vi "Recompile_all.vi"   [LabVIEW 2022 SP3]
uses:
  Anemometry Sub Vis/Globals/Constants_global.vi
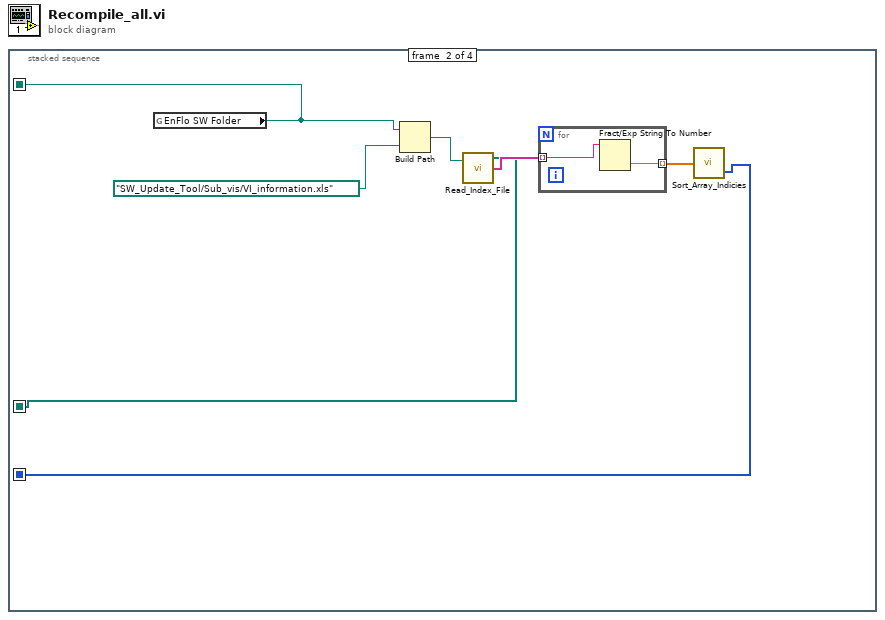
[diagram p0: block diagram]
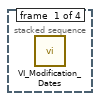
[diagram p2: hidden frame]
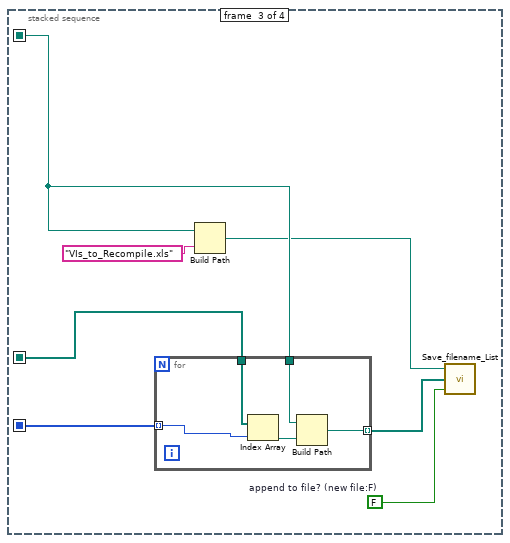
[diagram p3: hidden frame]
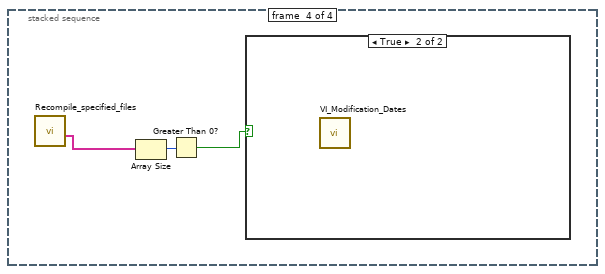
[diagram p4: hidden frame]
diagram:
  n1 = stacked-sequence {
    seq-local: [_ w3 _ _] -> [_ _ w15 _]
    seq-local: [_ w2 _ _] -> [_ _ w14 _]
    seq-local: [_ w1 _ _] -> [_ _ w13 _]
    frame #0 {
      n2 = call "VI_Modification_Dates.vi"() -> ()  [unwired: 1 out]
    }
    frame #1 {
      n3 = global read "Constants_global.vi" "EnFlo SW Folder"() -> (w1:path)
      n4 = Build Path(base path=w1, name or relative path=path "SW_Update_Tool/Sub_vis/VI_information.xls") -> (appended path=w6:path)
      n5 = call "Read_Index_File.vi"("Index Filename"=w6) -> ("Filenames"=w2:path[], "No of Sub vis"=w5:string[])  [unwired: 1 in, 1 out]
      n6 = for {
        tunnel: w5 -> [w8] mode=indexing
        tunnel: [w9] -> w4 mode=indexing
        n7 = Fract/Exp String To Number(string=w8) -> (number=w9:dbl)  [unwired: 4 out]
      }
      n8 = call "Sort_Array_Indicies.vi"("unsorted array"=w4) -> ("Sort Index"=w3:i32[])  [unwired: 1 out]
    }
    frame #2 {
      w10 = FALSE  # append to file? (new file:F)
      n9 = for {
        tunnel: w14 -> [w21]
        tunnel: w13 -> [w20]
        tunnel: w15 -> [w18] mode=indexing
        tunnel: [w17] -> w12 mode=indexing
        n10 = Index Array(array=w21, index=w18) -> (element=w19:path)
        n11 = Build Path(base path=w20, name or relative path=w19) -> (appended path=w17:path)
      }
      n12 = Build Path(base path=w13, name or relative path="VIs_to_Recompile.xls") -> (appended path=w11:path)
      n13 = call "Save_filename_List.vi"("append to file? (new file:F)"=w10, "Filename to save"=w12, "file path (dialog if empty)"=w11) -> ()  [unwired: 1 out]
    }
    frame #3 {
      n14 = call "Recompile_specified_files.vi"() -> ("Saved Vis paths Out"=w24:string[])  [unwired: 5 out]
      n15 = Array Size(array=w24) -> (size(s)=w23:i32)
      n16 = Greater Than 0?(x=w23) -> (x > 0?=w22:bool)
      n17 = case shown="True" w22 {
        frame False {
        }
        frame True {
          n18 = call "VI_Modification_Dates.vi"() -> ()  [unwired: 1 out]
        }
      }
    }
  }
